vi "Set Extended Identifier.vi"(8 "error in (no error)":errorcluster, 10 "Extended Identifier?":bool, 11 "CAN Frame in":refnum<class "CAN Frame.lvclass">) -> (0 "error out":errorcluster, 3 "CAN Frame out":refnum<class "CAN Frame.lvclass">)   [LabVIEW 2023, in "CAN Frame.lvclass"]
uses:
  CAN Frame.lvclass
  CAN Frame.lvclass/CAN Frame.ctl
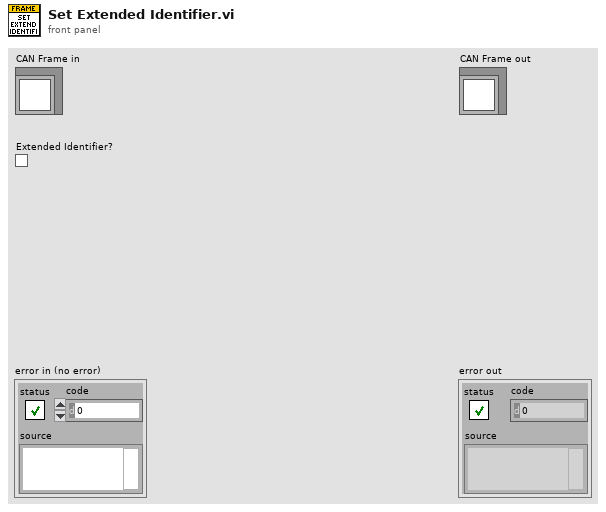
[diagram p1: front panel]
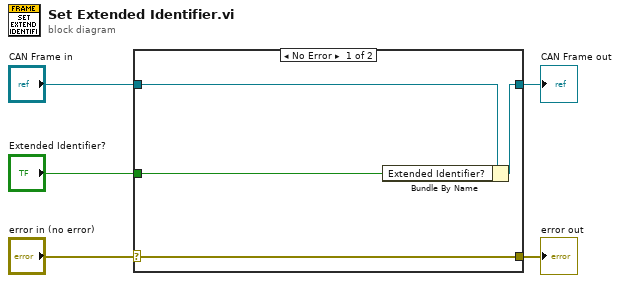
[diagram p0: block diagram]
diagram:
  n1 = case shown="No Error" "error in (no error)" {
    selector: "error in (no error)" -> [w9 w10]
    tunnel: [w9 w10] -> w4
    tunnel: [w7 w11] -> w2
    tunnel: "CAN Frame in" -> [w8 w11]
    tunnel: "Extended Identifier?" -> [w6 _]
    frame No Error {
      n2 = Bundle By Name(cluster=w8, "Extended Identifier?"=w6) -> (w7:refnum<class "CAN Frame.lvclass">)
    }
    frame Error {
    }
  }
  "error out" <- w4
  "CAN Frame out" <- w2
